vi "UpdateProgressBar.vi"(8 "error in (no error)":errorcluster, 9 "file name":string, 10 "current":i32, 11 "reference in":refnum<vi>) -> (0 "error out":errorcluster, 3 "reference out":refnum<vi>)   [LabVIEW 2017]
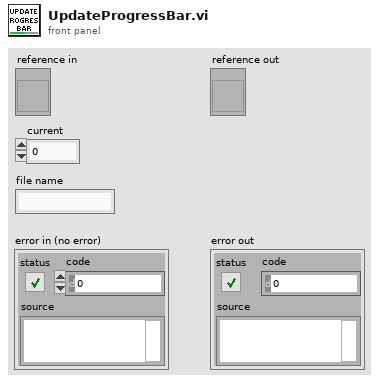
[diagram p1: front panel]
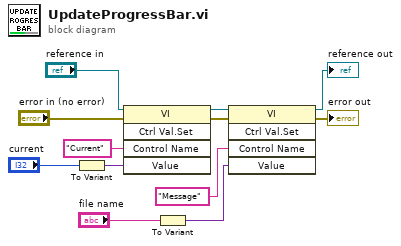
[diagram p0: block diagram]
diagram:
  n1 = To Variant(anything="current") -> (Variant=w8:variant)
  n2 = invoke class="VI" method="Ctrl Val.Set"(reference="reference in", error in="error in (no error)", "Control Name"="Current", "Value"=w8) -> (reference out=w10:refnum<vi>, error out=w5:errorcluster)  [unwired: 1 in, 3 out]
  n3 = To Variant(anything="file name") -> (Variant=w1:variant)
  n4 = invoke class="VI" method="Ctrl Val.Set"(reference=w10, error in=w5, "Control Name"="Message", "Value"=w1) -> (reference out=→"reference out":refnum<vi>, error out=→"error out":errorcluster)  [unwired: 1 in, 3 out]
